vi "Run Instrument Framework Test Suite.vi"   [LabVIEW 2019]
uses:
  <userlib>/LevyLab/RemoteControl/RemoteControl/Typedefs/RC Com Type--enum.ctl
  <userlib>/LevyLab/RemoteControl/RemoteControl/RemoteControl.lvclass
types:
  T1 = typedef "RemoteControl.lvclass/RC Com Type--enum.ctl" = enum16{"RC", "STM", "ZMQ"}
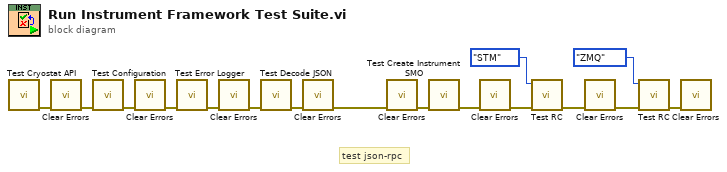
[diagram p0: block diagram]
diagram:
  # "test json-rpc"
  n1 = call "Test Cryostat API.vi"() -> ("error out"=w14:errorcluster)  [unwired: 11 in]
  n2 = call <vilib>:"Clear Errors.vi"("error in (no error)"=w14) -> ("error out"=w9:errorcluster)  [unwired: 5 in, 1 out]
  n3 = call "Test Configuration.vi"("error in (no error)"=w9) -> ("error out"=w8:errorcluster)  [unwired: 10 in]
  n4 = call <vilib>:"Clear Errors.vi"("error in (no error)"=w8) -> ("error out"=w4:errorcluster)  [unwired: 5 in, 1 out]
  n5 = call "Test Error Logger.vi"("error in (no error)"=w4) -> ("error out"=w3:errorcluster)  [unwired: 10 in]
  n6 = call <vilib>:"Clear Errors.vi"("error in (no error)"=w3) -> ("error out"=w2:errorcluster)  [unwired: 5 in, 1 out]
  n7 = call "Test Decode JSON.vi"("error in (no error)"=w2) -> ("error out"=w7:errorcluster)  [unwired: 10 in]
  n8 = call <vilib>:"Clear Errors.vi"("error in (no error)"=w7) -> ("error out"=w1:errorcluster)  [unwired: 5 in, 1 out]
  n9 = call <vilib>:"Clear Errors.vi"("error in (no error)"=w1) -> ("error out"=w10:errorcluster)  [unwired: 5 in, 1 out]
  n10 = call "Test Create Instrument SMO.vi"("error in (no error)"=w10) -> ("error out"=w12:errorcluster)  [unwired: 10 in]
  n11 = call <vilib>:"Clear Errors.vi"("error in (no error)"=w12) -> ("error out"=w11:errorcluster)  [unwired: 5 in, 1 out]
  n12 = call "Test RC.vi"("error in (no error)"=w11, "RC Type"=RC_Com_Type--enum."STM") -> ("error out"=w15:errorcluster)  [unwired: 9 in]
  n13 = call <vilib>:"Clear Errors.vi"("error in (no error)"=w15) -> ("error out"=w13:errorcluster)  [unwired: 5 in, 1 out]
  n14 = call "Test RC.vi"("error in (no error)"=w13, "RC Type"=RC_Com_Type--enum."ZMQ") -> ("error out"=w16:errorcluster)  [unwired: 9 in]
  n15 = call <vilib>:"Clear Errors.vi"("error in (no error)"=w16) -> ()  [unwired: 5 in, 2 out]
